vi "GV trigger AO and DO.vi"() -> ()   [LabVIEW 2017]
panel:
  out "AO/DO trig":bool
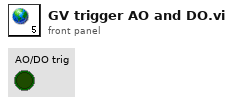
[diagram p1: front panel]
diagram:
